vi "LegendWDTWaveformGraph.vi"(8 "error in (no error)":errorcluster, 9 "Plot.Plot Name":string, 10 "Active Plot":i32, 11 "WFGraph (WDT) in":refnum<vi>) -> (0 "error out":errorcluster, 1 "Plot.Plot Name":string, 2 "Active Plot":i32, 3 "WFGraph (WDT) out":refnum<vi>)   [LabVIEW 2016, in "Instrument.Lockin.lvclass"]
uses:
  Instrument.Lockin.lvclass
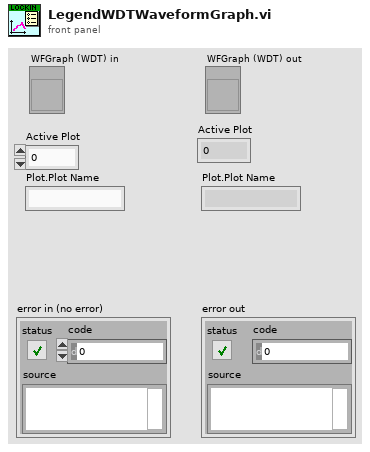
[diagram p1: front panel]
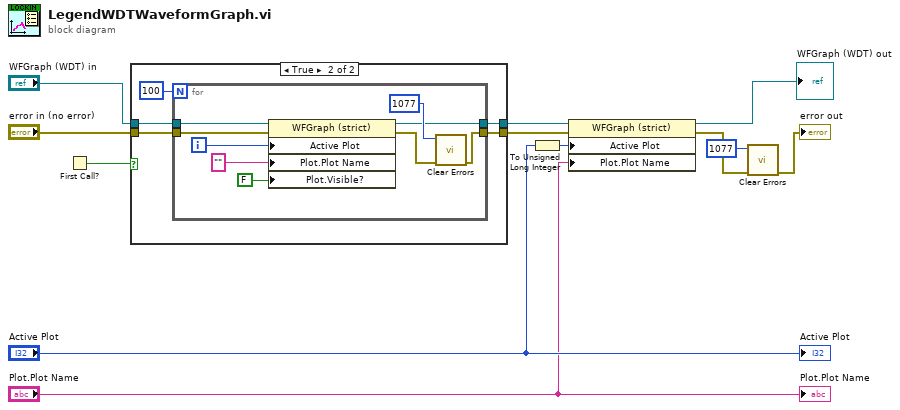
[diagram p0: block diagram]
diagram:
  n1 = First Call?() -> (First Call?: T/F=w4:bool)
  n2 = case shown="True" w4 {
    tunnel: "WFGraph (WDT) in" -> [w13 w16]
    tunnel: [w14 w19] -> w6
    tunnel: "error in (no error)" -> [w14 w18]
    tunnel: [w13 w15] -> w5
    frame False {
    }
    frame True {
      n3 = for {
        N: 100 -> [_]
        tunnel: w16 -> [w22]
        tunnel: [w26] -> w19
        tunnel: w18 -> [w21]
        tunnel: [w20] -> w15
        i -> [w25]
        n4 = property on="Property Node" class="WFGraph (strict)"(reference=w22, error in=w21, "Active Plot"=w25, "Plot.Plot Name"="" ("format string"), "Plot.Visible?"=FALSE ("Plot.Visible")) -> (reference out=w20:refnum<vi>, error out=w27:errorcluster)
        n5 = call <vilib>:"Clear Errors.vi"("error in (no error)"=w27, "specific error code to clear (0: all)"=1077) -> ("error out"=w26:errorcluster)  [unwired: 4 in, 1 out]
      }
    }
  }
  n6 = To Unsigned Long Integer(number="Active Plot") -> (unsigned 32bit integer=w7:u32)
  n7 = property on="Property Node" class="WFGraph (strict)"(reference=w5, error in=w6, "Active Plot"=w7, "Plot.Plot Name"="Plot.Plot Name") -> (reference out=→"WFGraph (WDT) out":refnum<vi>, error out=w11:errorcluster)
  n8 = call <vilib>:"Clear Errors.vi"("error in (no error)"=w11, "specific error code to clear (0: all)"=1077) -> ("error out"=→"error out":errorcluster)  [unwired: 4 in, 1 out]
  "Active Plot" <- "Active Plot"
  "Plot.Plot Name" <- "Plot.Plot Name"
